vi "Configure System Date.vi"(7 "Day (01)":i32=1, 8 "error in (no error)":errorcluster, 9 "Month (01)":i32=1, 10 "Year (2023)":i32=2023, 11 "VISA resource name":refnum<visa-resource-name>) -> (0 "error out":errorcluster, 3 "VISA resource name out":refnum<visa-resource-name>)   [LabVIEW 2020, in "Rohde&Schwarz CMXP Base.lvlib"]
doc: "Sets the UTC date of the operating system calendar.\n\nAttribute:\n-\n\nRemote-control command:\nSYSTem:DATE[:UTC]"
uses:
  <instrlib>/Rohde&Schwarz CMXP Base/Rohde&Schwarz CMXP Base.lvlib
  <instrlib>/Rohde&Schwarz CMXP Base/Private/rsidr_core.llb/rsidr_core.lvlib
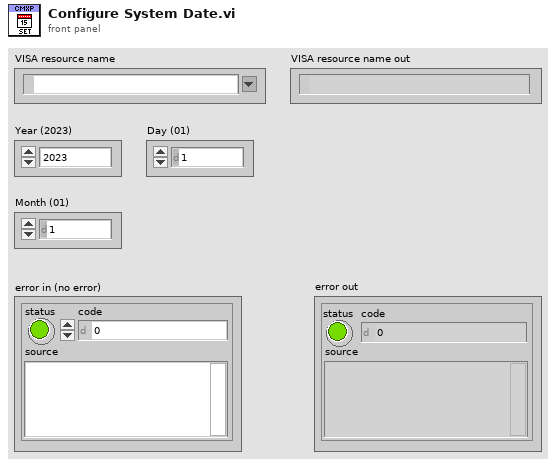
[diagram p1: front panel]
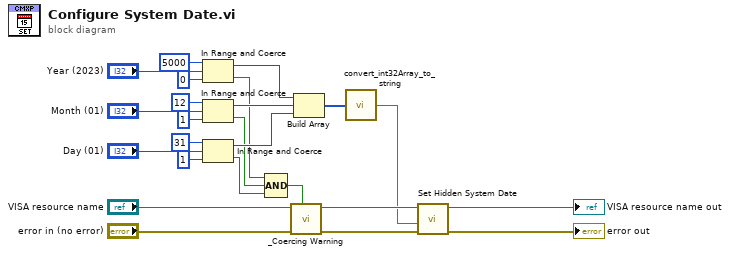
[diagram p0: block diagram]
diagram:
  n1 = In Range and Coerce(upper limit=5000, x="Year (2023)", lower limit=0) -> (coerced(x)=w12:i32, In Range?=w2:bool)
  n2 = In Range and Coerce(upper limit=12, x="Month (01)", lower limit=1) -> (coerced(x)=w13:i32, In Range?=w3:bool)
  n3 = In Range and Coerce(upper limit=31, x="Day (01)", lower limit=1) -> (coerced(x)=w14:i32, In Range?=w4:bool)
  n4 = Compound Arithmetic op=AND(w2, w3, w4) -> (w6:bool)
  n5 = call <instrlib>:"_Coercing Warning.vi"("In Range?"=w6, "error in (no error)"="error in (no error)", "VISA resource name"="VISA resource name") -> ("error out"=w9:errorcluster, "VISA resource name out"=w10:refnum<visa-resource-name>)  [unwired: 7 in]
  n6 = Build Array(w12, w13, w14) -> (w11:i32[])
  n7 = call <instrlib>:"convert_int32Array_to_string.vi"("I32 array in"=w11) -> ("string out"=w1:string)  [unwired: 4 in]
  n8 = call "Set Hidden System Date"("error in (no error)"=w9, "Hidden System Date ()"=w1, "instrument handle"=w10) -> ("error out"=→"error out":errorcluster, "instrument handle out"=→"VISA resource name out":refnum<visa-resource-name>)  [unwired: 7 in]
